vi "WPI_DefaultPWMConstants.vi"(0 "DIO Loop Timing (ticks)":u16=261) -> (14 "defaultPWMPeriod":u16=774, 15 "defaultMinPWMHigh":u16=102, 16 "defaultPWMDisabled":u16)   [LabVIEW 2017]
doc: "This software is licensed. Open the labview\\readme\\WPI Robotics Library Open Source License.txt file for more information."
panel:
  # "This VI is Subroutine"
  # "404 with new I/O node"
  # "Taken from WPI LabVIEW C code PWM.h back in 2008... the values are obsolete for roboRIO,\nthough the concepts hold.\n/**\n\t * kDefaultPwmPeriod is \"ticks\" where each tick is 6.525us\n\t * 20ms periods (50 Hz) are the \"safest\" setting in that this works for all devices\n\t * 20ms periods seem to be desirable for Vex Motors\n\t * 20ms periods are the specified period for HS-322HD servos, but work reliably down\n\t *      to 10.0 ms; starting at about 8.5ms, the servo sometimes hums and get hot;\n\t *      by 5.0ms the hum is nearly continuous\n\t * 10ms periods work well for Victor 884\n\t * 5ms periods allows higher update rates for Luminary Micro Jaguar speed controllers\n\t * \n\t * This is the 1x period (5ms).  In hardware, the period scaling is implemented as an\n\t *   output squelch to get longer periods for old devices.\n\t * Set to 5.05 ms period / 6.525us clock = 774\n\t */"
  # "/**\n\t * kDefaultMinPwmHigh is \"ticks\" where each tick is 6.525us\n\t * There are 127 pwm values less than the center, so...\n\t * The minimum output pulse length is 1.5ms - 127 * 6.525us = 0.671ms\n\t * 0.671ms / 6.525us per tick = 103\n\t */"
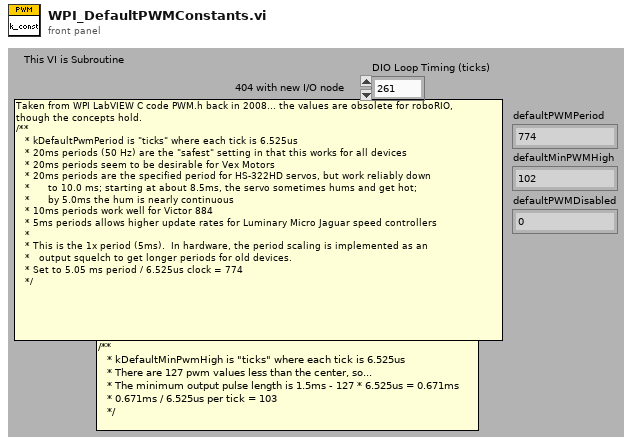
[diagram p1: front panel]
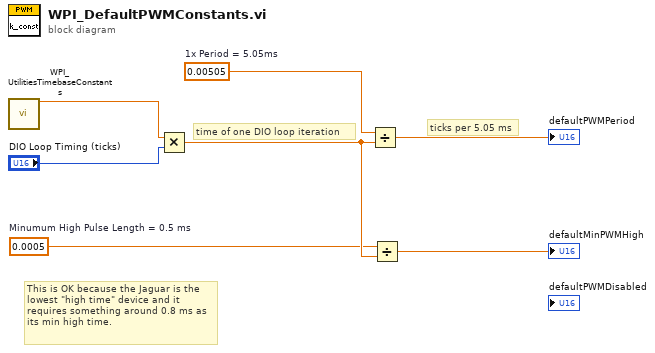
[diagram p0: block diagram]
diagram:
  w2 = 0.0005  # Minumum High Pulse Length = 0.5 ms
  w4 = 0.00505  # 1x Period = 5.05ms
  # "This is OK because the Jaguar is the lowest \"high time\" device and it requires something around 0.8 ms as its min high time."
  # "ticks per 5.05 ms"
  # "time of one DIO loop iteration"
  n1 = call <vilib>:"WPI_UtilitiesTimebaseConstants.vi"() -> ("40 MHz FPGA clock"=w1:dbl)  [unwired: 13 in, 2 out]
  n2 = Multiply(x=w1, y="DIO Loop Timing (ticks)") -> (x*y=w6:dbl)
  n3 = Divide(x=w4, y=w6) -> (x/y=→"defaultPWMPeriod":dbl)
  n4 = Divide(x=w2, y=w6) -> (x/y=→"defaultMinPWMHigh":dbl)
